vi "SAACPTraceRead.vi"(7 "RetValBufferSize":i32=2048 caption="RetValBufferSize (2048)", 8 "error in (no error)":errorcluster {"code" format="%.0x"}, 9 "MaxTime":i32=1000 caption="MaxTime (ms)" format="%#.0f", 10 "RepCapIdentifier":string="ACP_Results" caption="RepCapIdentifier (ACP_Results)", 11 "instrument handle":refnum<k15>) -> (0 "error out":errorcluster {"code" format="%.0x"}, 1 "RetValActualSize":i32, 2 "RetVal":dbl[](array[numeric]) format="%.2p", 3 "instrument handle out":refnum<k15>)   [LabVIEW 2009, in "Keysight XSAn.lvlib"]
doc: "Initiates the measurement and puts valid data into the output buffer.\n\nSupported Models: M9290A, N8973B, N8974B, N8975B, N8976B, N9000A, N9000B, N9010A, N9010B, N9020A, N9020B, N9030A, N9030B, N9038A, N9040B, N9041B, SPN9003A, SPN9026A"
uses:
  <instrlib>/Keysight XSAn/Keysight XSAn.lvlib
  AgXSAn.dll
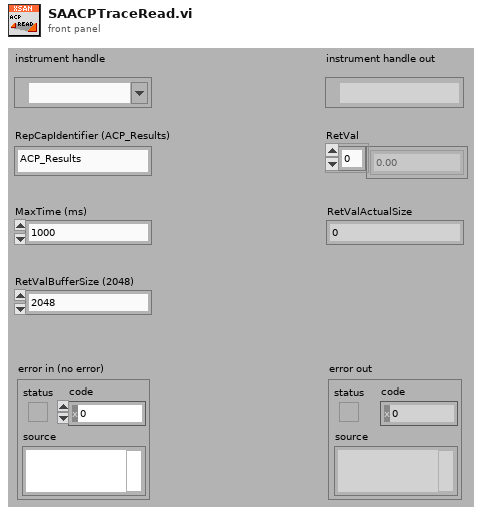
[diagram p1: front panel]
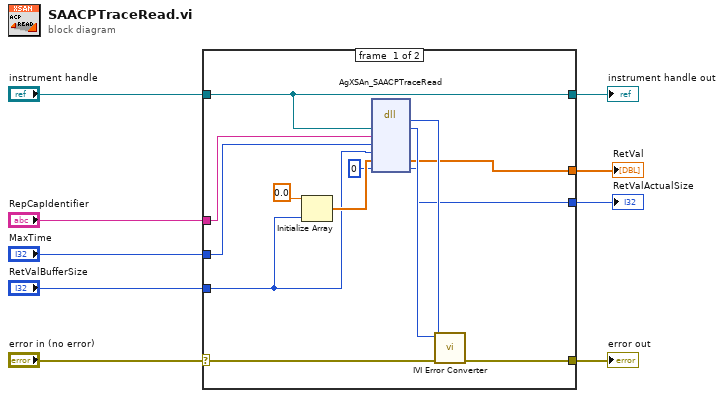
[diagram p0: block diagram]
diagram:
  n1 = case shown="No Error" "error in (no error)" {
    selector: "error in (no error)" -> [w20 w24]
    tunnel: [w19 w24] -> w9
    tunnel: "instrument handle" -> [w11 w23]
    tunnel: "RepCapIdentifier" -> [w18 _]
    tunnel: "MaxTime" -> [w17 _]
    tunnel: "RetValBufferSize" -> [w10 _]
    tunnel: [w14 _] -> w3
    tunnel: [w12 _] -> w2
    tunnel: [w11 w23] -> w1
    frame #0 {
      n2 = Initialize Array(0.0 ("element"), w10) -> (w16:dbl[])
      n3 = dll-call lib="AgXSAn**.dll" fn="AgXSAn_SAACPTraceRead"("Vi"=w11, "RepCapIdentifier"=w18, "MaxTime"=w17, "RetValBufferSize"=w10, "RetVal"=w16, "RetValActualSize"=0) -> (w21:i32, "Vi"=w22:u32, "RetVal"=w14:dbl[], "RetValActualSize"=w12:i32)  [unwired: 6 in, 2 out]
      n4 = call <instrlib>:"IVI Error Converter.vi"("error in (no error)"=w20, "IVI error code (0)"=w21, "instrument handle"=w22) -> ("error out"=w19:errorcluster)  [unwired: 7 in, 1 out]
    }
    frame #1 {
    }
  }
  "error out" <- w9
  "instrument handle out" <- w1
  "RetVal" <- w3
  "RetValActualSize" <- w2
